vi "Test Source Path in Error Source.vi"(8 "error in (no error)":errorcluster) -> (0 "error out":errorcluster)   [LabVIEW 2020]
uses:
  src/Deserializer/JSON Deserializer/JSON Deserializer.lvclass
  src/Deserializer/JSON Deserializer/JSON Deserializer.lvclass/JSON Deserializer.ctl
  <vilib>/addons/_JKI Toolkits/Caraya/classes/Assert/Assert True.vi
  <vilib>/regexp/Match Regular Expression.xnode
  <vilib>/addons/_JKI Toolkits/Caraya/classes/Test/Test.lvclass
  src/JKI JSON Serialization.lvlib
  <vilib>/addons/_JKI Toolkits/Caraya/classes/Assert/Assert.lvclass
panel:
  out "Array":errorcluster[](array[cluster])
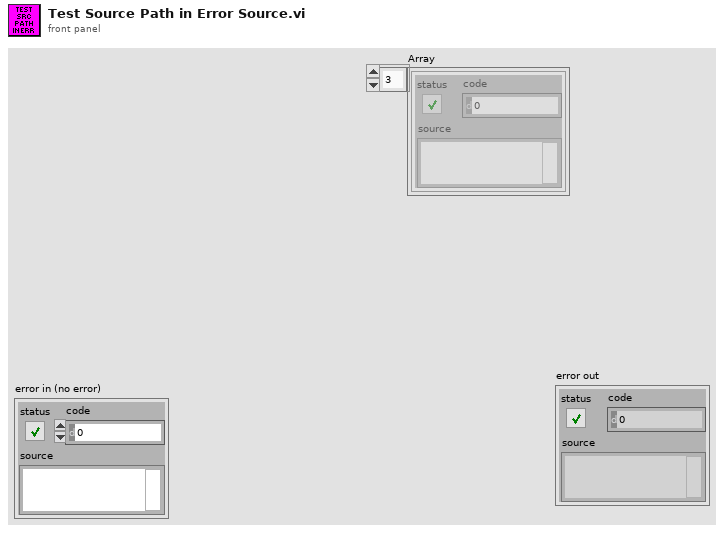
[diagram p1: front panel]
types:
  T1 = cluster{"test label":string, "source path":string, "input json":string, "error match":string}[]
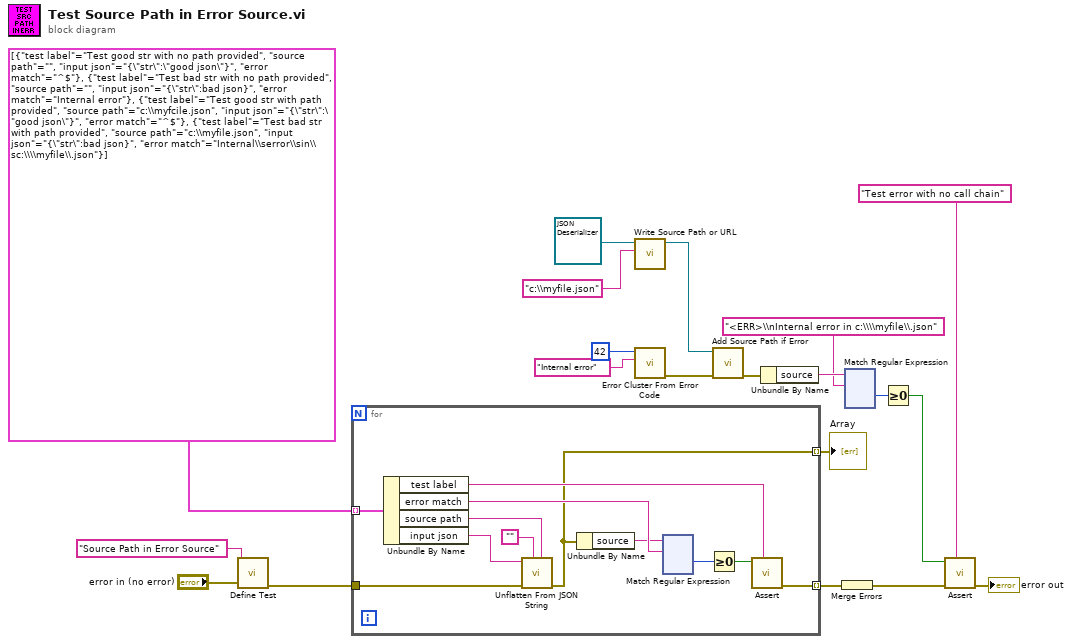
[diagram p0: block diagram]
diagram:
  n1 = call <vilib>:"Define Test.vi"("error in (no error)"="error in (no error)", "Label (VI Title)"="Source Path in Error Source") -> ("error out"=w17:errorcluster)  [unwired: 8 in, 1 out]
  n2 = for {
    tunnel: w17 -> [w32]
    tunnel: [w31] -> w18 mode=indexing
    tunnel: T1 [{"test label"="Test good str with no path provided", "source path"="", "input json"="{\"str\":\"good json\"}", "error match"="^$"}, {"test label"="Test bad str with no path provided", "source path"="", "input json"="{\"str\":bad json}", "error match"="Internal error"}, {"test label"="Test good str with path provided", "source path"="c:\\myfcile.json", "input json"="{\"str\":\"good json\"}", "error match"="^$"}, {"test label"="Test bad str with path provided", "source path"="c:\\myfile.json", "input json"="{\"str\":bad json}", "error match"="Internal\\serror\\sin\\sc:\\\\myfile\\.json"}] -> [w30] mode=indexing
    tunnel: [w21] -> w15 mode=indexing
    n3 = Unbundle By Name(w30) -> ("test label"=w29:string, "error match"=w25:string, "source path"=w28:string, "input json"=w27:string)
    n4 = call "Unflatten From JSON String.vi"("Source Path or URL"=w28, "Type and Defaults"="", "error in (no error)"=w32, "JSON String"=w27) -> ("error out"=w21:errorcluster)  [unwired: 6 in, 1 out]
    n5 = Unbundle By Name(w21) -> ("source"=w22:string)
    n6 = xnode ("Match Regular Expression")("input string"=w22, "regular expression"=w25) -> ("offset past match"=w24:i32)  [unwired: 4 in, 4 out]
    n7 = Greater Or Equal To 0?(x=w24) -> (x >= 0?=w23:bool)
    n8 = call-poly <vilib>:"Assert.vi"("Label"=w29, "True?"=w23) -> ("error out"=w31:errorcluster)  [unwired: 8 in, 1 out]
  }
  "Array" <- w15
  n9 = call "Write Source Path or URL.vi"("Source Path or URL"="c:\\myfile.json" ("source path"), "JSON Deserializer in"=refnum<class "JSON Deserializer.lvclass"> refnum ("JKI JSON Serialization.lvlib:JSON Deserializer.lvclass")) -> ("JSON Deserializer out"=w9:refnum<class "JSON Deserializer.lvclass">)  [unwired: 8 in, 1 out]
  n10 = call <vilib>:"Error Cluster From Error Code.vi"("error message (\"\")"="Internal error" ("error message (\"\")"), "error code (0)"=42) -> ("error out"=w11:errorcluster)  [unwired: 7 in]
  n11 = call-dynamic "Add Source Path if Error.vi"("error in (no error)"=w11, "JSON Deserializer in"=w9) -> ("error out"=w5:errorcluster)  [unwired: 8 in, 1 out]
  n12 = Unbundle By Name(w5) -> ("source"=w3:string)
  n13 = Merge Errors(w18) -> (w14:errorcluster)
  n14 = xnode ("Match Regular Expression")("input string"=w3, "regular expression"="<ERR>\\nInternal error in c:\\\\myfile\\.json" ("Label")) -> ("offset past match"=w4:i32)  [unwired: 4 in, 4 out]
  n15 = Greater Or Equal To 0?(x=w4) -> (x >= 0?=w2:bool)
  n16 = call-poly <vilib>:"Assert.vi"("Label"="Test error with no call chain", "error in (no error)"=w14, "True?"=w2) -> ("error out"=→"error out":errorcluster)  [unwired: 7 in, 1 out]
